vi "DHE_SetModifiers.vi"(2 "DHE_Modifiers":string) -> ()   [LabVIEW 2016]
uses:
  private/vis/DHE_GBLDriverVariables.vi
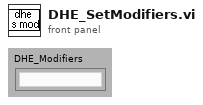
[diagram p1: front panel]
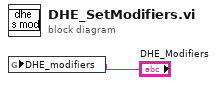
[diagram p0: block diagram]
diagram:
  n1 = global write "DHE_GBLDriverVariables.vi" "DHE_modifiers"("DHE_Modifiers") -> ()
